vi "Str to Connstr Cluster.vi"(11 "Connstr":string) -> (3 "output cluster":T1)   [LabVIEW 2014]
uses:
  Database/Ctr/Constr.ctl
panel:
  out "Array":string[](array[string])
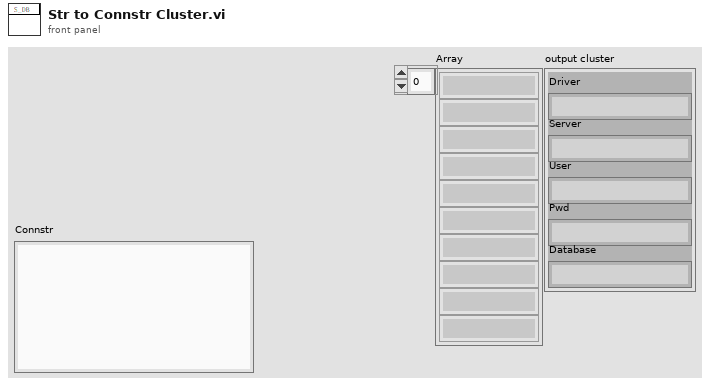
[diagram p1: front panel]
types:
  T1 = typedef "Constr.ctl" = cluster{"Driver":string, "Server":string, "User":string, "Pwd":string, "Database":string}
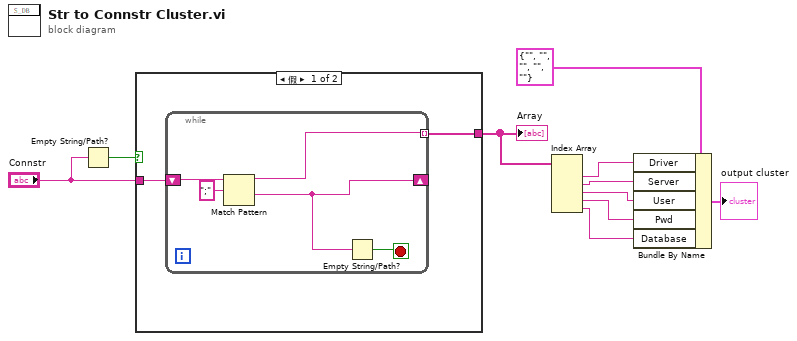
[diagram p0: block diagram]
diagram:
  n1 = Empty String/Path?(string/path="Connstr") -> (empty?=w9:bool)
  n2 = case shown="假" w9 {
    tunnel: [w12 _] -> w8
    tunnel: "Connstr" -> [w11 _]
    frame False {
      n3 = while {
        shift-right: [w14] -> _
        shift-left: w11 -> [w17]
        tunnel: [w13] -> w12 mode=indexing
        stop <- w15 stop-if-true
        n4 = Match Pattern(string=w17, regular expression=";") -> (before substring=w13:string, after substring=w14:string)  [unwired: 1 in, 2 out]
        n5 = Empty String/Path?(string/path=w14) -> (empty?=w15:bool)
      }
    }
    frame True {
    }
  }
  "Array" <- w8
  n6 = Index Array(array=w8) -> (element #1=w6:string, element #2=w5:string, element #3=w4:string, element #4=w3:string, element #5=w2:string)  [unwired: 5 in]
  n7 = Bundle By Name(cluster=T1 {"Driver"="", "Server"="", "User"="", "Pwd"="", "Database"=""} ("Constr"), "Driver"=w6, "Server"=w5, "User"=w4, "Pwd"=w3, "Database"=w2) -> (→"output cluster":T1)
